vi "Write Alarms_.vi"(8 "error in (no error)":errorcluster, 10 "Alarms?":bool, 11 "Filter Wheel in":refnum<class "Filter Wheel.lvclass">) -> (0 "error out":errorcluster, 3 "Filter Wheel out":refnum<class "Filter Wheel.lvclass">)   [LabVIEW 2021, in "Filter Wheel.lvclass"]
uses:
  Filter Wheel.lvclass
  Filter Wheel.lvclass/Filter Wheel.ctl
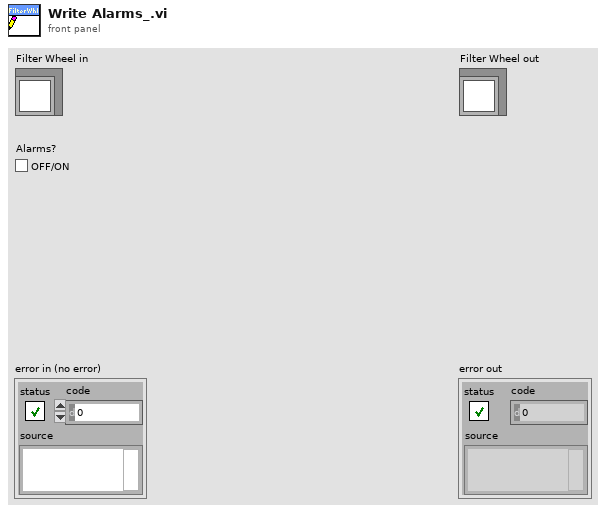
[diagram p1: front panel]
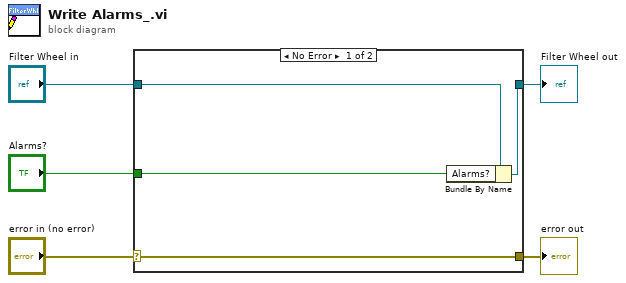
[diagram p0: block diagram]
diagram:
  n1 = case shown="No Error" "error in (no error)" {
    selector: "error in (no error)" -> [w9 w10]
    tunnel: [w9 w10] -> w4
    tunnel: [w7 w11] -> w2
    tunnel: "Filter Wheel in" -> [w8 w11]
    tunnel: "Alarms?" -> [w6 _]
    frame No Error {
      n2 = Bundle By Name(cluster=w8, "Alarms?"=w6) -> (w7:refnum<class "Filter Wheel.lvclass">)
    }
    frame Error {
    }
  }
  "error out" <- w4
  "Filter Wheel out" <- w2
